vi "Launch Server.vi"(0 "WebSocket Server Manager in":refnum<class "WebSocket Server Manager.lvclass">, 2 "Receive Server Enqueuer Handler":refnum<class "WebSocket Server-Service Enqueuer Msg.lvclass">, 5 "Listener Settings":T1={"resolve remote address (T)"=TRUE, "timeout ms (-1)"=-1, "net address"=0, "port"=6163}, 7 "Handshake timeout (5000 ms)":i32=5000, 9 "Subscriber Enqueuer":refnum<class "Message Enqueuer.lvclass">, 11 "error in (no error)":errorcluster) -> (4 "WebSocket Server Manager out":refnum<class "WebSocket Server Manager.lvclass">, 15 "error out":errorcluster)   [LabVIEW 2016, in "WebSocket Actors.lvlib" / "WebSocket Server Manager.lvclass"]
doc: "This method launches a server leistening on at a specified port and interface address as detailed in the \"Listener Settings\" input. If the server is already running at that port or on the specified interface the method sends just the server enqueuer ro the client. If the server is not running it will be launched."
uses:
  WebSocket Server Manager.lvclass
  C:/Program Files (x86)/National Instruments/LabVIEW 2016/vi.lib/ActorFramework/Actor/Actor.lvclass
  WebSocket Server/typedefs/Listener Settings.ctl
  <vilib>/ActorFramework/Message Enqueuer/Message Enqueuer.lvclass
  Abstract Messages/WebSocket Server-Service Enqueuer Msg/WebSocket Server-Service Enqueuer Msg.lvclass
  C:/Program Files (x86)/National Instruments/LabVIEW 2016/vi.lib/ActorFramework/Message/Message.lvclass
  WebSocket Server Manager.lvclass/WebSocket Server Manager.ctl
  WebSocket Server/WebSocket Server.lvclass
  WebSocket Server/WebSocket Server.lvclass/WebSocket Server.ctl
  Abstract Messages/WebSocket Server-Service Enqueuer Msg/WebSocket Server-Service Enqueuer Msg.lvclass/WebSocket Server-Service Enqueuer Msg.ctl
  <vilib>/ActorFramework/Message Enqueuer/Message Enqueuer.lvclass/Message Enqueuer.ctl
  WebSocket Server/properties/Write Handshake timeout (5000 ms).vi
  WebSocket Server/properties/Write Listener Settings.vi
  WebSocket Server/properties/Write URI.vi
  <vilib>/ActorFramework/Message Enqueuer/Enqueue.vi
  <vilib>/Utility/error.llb/Error Cluster From Error Code.vi
  <vilib>/ActorFramework/Message Priority Queue/Priority Enqueue.vi
  <vilib>/ErrorRing/Error Ring.xnode
  <vilib>/ActorFramework/Actor/Actor.lvclass
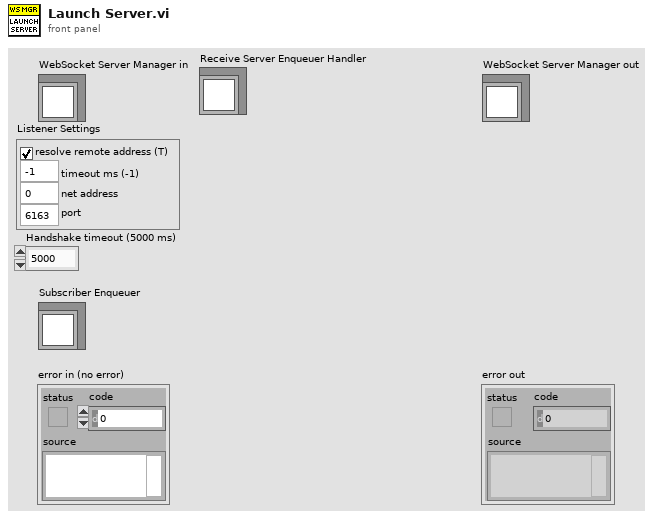
[diagram p1: front panel]
types:
  T1 = typedef "WebSocket Actors.lvlib/WebSocket Server.lvclass/Listener Settings.ctl" = cluster{"resolve remote address (T)":bool, "timeout ms (-1)":i32, "net address":u32, "port":u16}
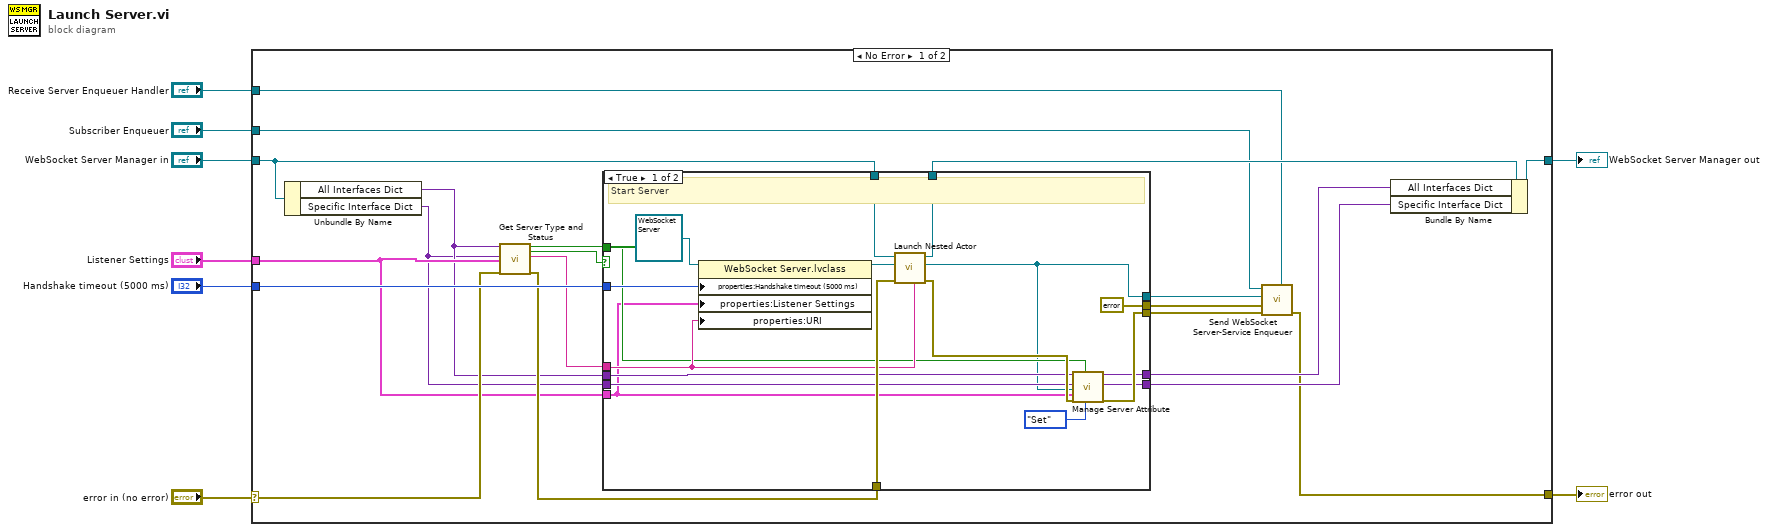
[diagram p0: block diagram]
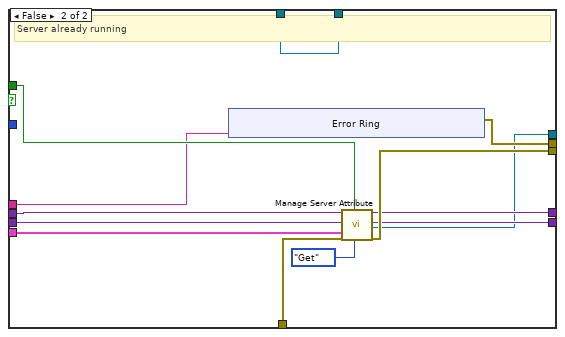
[diagram p2: hidden frame]
diagram:
  n1 = case shown="No Error" "error in (no error)" {
    selector: "error in (no error)" -> [w24 w68]
    tunnel: [w16 w68] -> w7
    tunnel: [w28 w67] -> w5
    tunnel: "WebSocket Server Manager in" -> [w27 w67]
    tunnel: "Handshake timeout (5000 ms)" -> [w25 _]
    tunnel: "Listener Settings" -> [w12 _]
    tunnel: "Subscriber Enqueuer" -> [w21 _]
    tunnel: "Receive Server Enqueuer Handler" -> [w15 _]
    frame No Error {
      n2 = Unbundle By Name(w27) -> ("All Interfaces Dict"=w11:variant, "Specific Interface Dict"=w9:variant)
      n3 = call "Get Server Type and Status.vi"("All Interfaces Dict"=w11, "Specific Interface Dict in"=w9, "Listener Settings"=w12, "error in (no error)"=w24) -> ("Is \"All Interface\" Server"=w19:bool, "Server Running"=w23:bool, "Server URI"=w14:string, "error out"=w13:errorcluster)  [unwired: 12 in]
      n4 = case shown="True" w23 {
        tunnel: w27 -> [w44 w59]
        tunnel: [w43 w59] -> w26
        tunnel: w25 -> [w42 _]
        tunnel: w12 -> [w29 w49]
        tunnel: w13 -> [w41 w57]
        tunnel: w14 -> [w39 w47]
        tunnel: [w36 w54] -> w22
        tunnel: [w30 w50] -> w10
        tunnel: [errorcluster {"status"=FALSE, "code"=0, "source"=""} ("error out") w58] -> w20
        tunnel: w19 -> [w31 w48]
        tunnel: w11 -> [w33 w56]
        tunnel: [w34 w53] -> w18
        tunnel: [w35 w52] -> w17
        tunnel: w9 -> [w32 w55]
        frame True {
          # "Start Server"
          n5 = property class="WebSocket Server.lvclass"(reference=refnum<class "WebSocket Server.lvclass"> refnum ("WebSocket Actors.lvlib:WebSocket Server.lvclass"), "properties:Handshake timeout (5000 ms)"=w42, "properties:Listener Settings"=w29, "properties:URI"=w39) -> (reference out=w45:refnum<class "WebSocket Server.lvclass">)  [unwired: 1 in, 1 out]
          n6 = call <vilib>:"Launch Nested Actor.vi"("Debug Alias"=w39, "error in (no error)"=w41, "Nested Actor"=w45, "Caller Actor in"=w44) -> ("error out"=w37:errorcluster, "Nested Actor's Enqueuer"=w30:refnum<class "Message Enqueuer.lvclass">, "Caller Actor out"=w43:refnum<class "WebSocket Server Manager.lvclass">)  [unwired: 5 in]
          n7 = call "Manage Server Attribute.vi"("All Interfaces Dict in"=w33, "Specific Interface Dict in"=w32, "Message Enqueuer in"=w30, "Listener Settings"=w29, "error in (no error)"=w37, "Is \"All Interface\" Server"=w31, "Action"=enum16{"Set", "Get", "Delete"}."Set") -> ("All Interfaces Dict out"=w35:variant, "Specific Interface Dict out"=w34:variant, "error out"=w36:errorcluster)  [unwired: 9 in, 1 out]
        }
        frame False {
          # "Server already running"
          n8 = xnode "Error Ring"("parameter 0"=w47) -> ("error out"=w58:errorcluster)
          n9 = call "Manage Server Attribute.vi"("All Interfaces Dict in"=w56, "Specific Interface Dict in"=w55, "Listener Settings"=w49, "error in (no error)"=w57, "Is \"All Interface\" Server"=w48, "Action"=enum16{"Set", "Get", "Delete"}."Get") -> ("All Interfaces Dict out"=w52:variant, "Specific Interface Dict out"=w53:variant, "Message Enqueuer out"=w50:refnum<class "Message Enqueuer.lvclass">, "error out"=w54:errorcluster)  [unwired: 10 in]
        }
      }
      n10 = call "Send WebSocket Server-Service Enqueuer.vi"("Receive Service/Server Enqueuer Handler"=w15, "error in (no error)"=w22, "Error"=w20, "WebSocket Server/Service Enqueuer"=w10, "Message Enqueuer"=w21) -> ("error out"=w16:errorcluster)  [unwired: 5 in, 1 out]
      n11 = Bundle By Name(cluster=w26, "All Interfaces Dict"=w17, "Specific Interface Dict"=w18) -> (w28:refnum<class "WebSocket Server Manager.lvclass">)
    }
    frame Error {
    }
  }
  "error out" <- w7
  "WebSocket Server Manager out" <- w5
